vi "MCP23S17 Read REG.vi"(8 "error in (no error)":errorcluster, 10 "Addr":T1 items=["Addr-0"=0, "Addr-1"=4, "Addr-2"=2, "Addr-3"=6, "Addr-4"=1, "Addr-5"=5, "Addr-6"=3, "Addr-7"=7], 11 "handle":u32 format="%08x") -> (0 "error out":errorcluster, 1 "REG B":u16, 2 "REG A":u16, 3 "handle out":u32, 5 "buffer out B":string, 7 "buffer out A":string)   [LabVIEW 2018]
uses:
  PROJEKT/NIKO/Labview/Niko V4/FTDI SPI/Ctl/Sub Addr.ctl
  PROJEKT/NIKO/Labview/Niko V6_A/FTDI SPI/libMPSSE-SPI.lvlib
panel:
  in  "Array U8 2":u8[](array[numeric])=[64, 18, 0, 128, 0, 0, 0, 0, 0, 0] format="%x"
  out "string":string
  in  "Array U8":u8[](array[numeric])=[64, 18, 0, 128, 0, 0, 0, 0, 0, 0] format="%x"
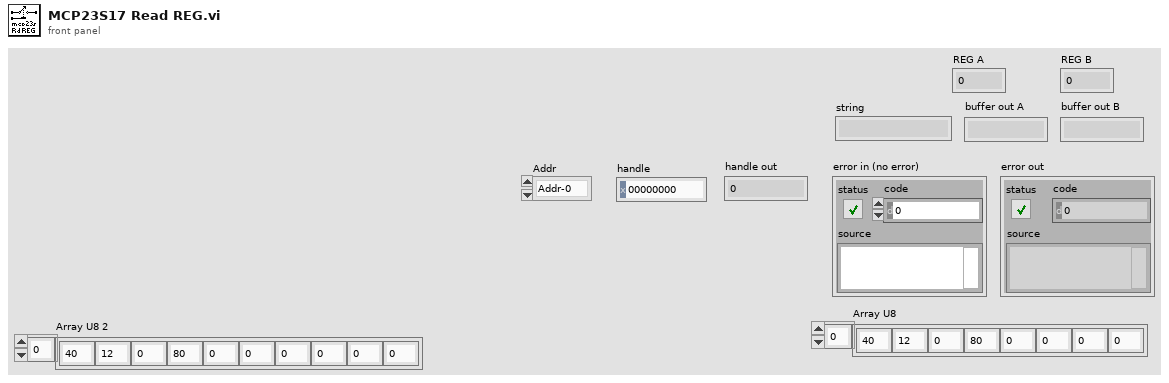
[diagram p1: front panel]
types:
  T1 = typedef "Sub Addr.ctl" = u16
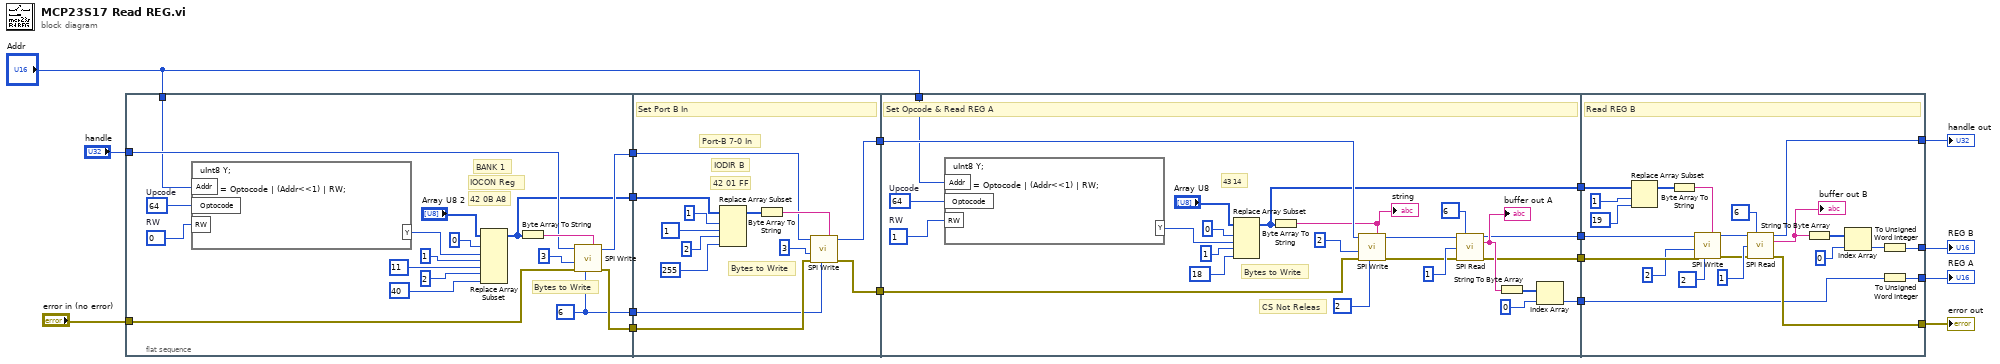
[diagram p0: block diagram]
diagram:
  n1 = flat-sequence {
    tunnel: [w20] -> w7
    tunnel: [w24] -> w6
    tunnel: "handle" -> [w23]
    tunnel: "Addr" -> [w22]
    tunnel: "error in (no error)" -> [w21]
    tunnel: [w19] -> w2
    tunnel: [w18] -> w1
    tunnel: [w41] -> w9
    tunnel: [w40] -> w8
    tunnel: w7 -> [w39]
    tunnel: w6 -> [w38]
    tunnel: w2 -> [w37]
    tunnel: w1 -> [w36]
    tunnel: [w53] -> w16
    tunnel: [w52] -> w15
    tunnel: [w51] -> w14
    tunnel: [w50] -> w13
    tunnel: w9 -> [w68]
    tunnel: w8 -> [w65]
    tunnel: "Addr" -> [w49]
    tunnel: [w92] -> w17
    tunnel: [w91] -> w12
    tunnel: w16 -> [w86]
    tunnel: w15 -> [w82]
    tunnel: w14 -> [w80]
    tunnel: w13 -> [w75]
    tunnel: [w74] -> w11
    tunnel: [w73] -> w10
    frame #0 {
      w35 = u8 64  # Upcode
      w34 = u8 0  # RW
      w18 = u8 6
      # "BANK 1"
      # "IOCON Reg"
      # "Bytes to Write"
      # "42 0B A8"
      n2 = formula code="uInt8 Y;\n      \n    Y = Optocode | (Addr<<1) | RW;"("Addr"=w22, "Optocode"=w35, "RW"=w34) -> ("Y"=w26:u8)
      n3 = Replace Array Subset(array="Array U8 2", new element #1=w26, index #1=0 ("index"), new element #2=u8 11, index #2=u8 1 ("new element/subarray"), new element #3=u8 40, index #3=2 ("index")) -> (w19:u8[])
      n4 = Byte Array To String(unsigned byte array=w19) -> (string=w31:string)
      n5 = call "SPI Write.vi"("buffer"=w31, "options"=w18, "error in (no error)"=w21, "Bytes To Send"=u32 3, "handle"=w23) -> ("error out"=w20:errorcluster, "handle out"=w24:u32)  [unwired: 4 in, 1 out]
    }
    frame #1 {
      # "IODIR B"
      # "Port-B 7-0 In"
      # "Bytes to Write"
      # "42 01 FF"
      # "Set Port B In"
      n6 = Replace Array Subset(array=w37, new element #1=u8 1, index #1=1 ("index"), new element #2=u8 255, index #2=2 ("index")) -> (w45:u8[])
      n7 = Byte Array To String(unsigned byte array=w45) -> (string=w44:string)
      n8 = call "SPI Write.vi"("buffer"=w44, "options"=w36, "error in (no error)"=w39, "Bytes To Send"=u32 3, "handle"=w38) -> ("error out"=w40:errorcluster, "handle out"=w41:u32)  [unwired: 4 in, 1 out]
    }
    frame #2 {
      w61 = u8 64  # Upcode
      w62 = u8 1  # RW
      # "CS Not Releas"
      # "Bytes to Write"
      # "43 14"
      # "Set Opcode & Read REG A"
      n9 = formula code="uInt8 Y;\n      \n    Y = Optocode | (Addr<<1) | RW;"("Addr"=w49, "Optocode"=w61, "RW"=w62) -> ("Y"=w71:u8)
      n10 = Replace Array Subset(array="Array U8", new element #1=w71, index #1=0 ("index"), new element #2=u8 18, index #2=u8 1 ("new element/subarray")) -> (w53:u8[])
      n11 = Byte Array To String(unsigned byte array=w53) -> (string=w67:string)
      "string" <- w67
      n12 = call "SPI Write.vi"("buffer"=w67, "options"=u8 2, "error in (no error)"=w65, "Bytes To Send"=u32 2, "handle"=w68) -> ("error out"=w57:errorcluster, "handle out"=w58:u32)  [unwired: 4 in, 1 out]
      n13 = call "SPI Read.vi"("handle"=w58, "options"=u8 6, "sizeToTransfer"=u32 1, "error in (no error)"=w57) -> ("handle out"=w52:u32, "buffer out"=w54:string, "error out"=w51:errorcluster)  [unwired: 7 in, 2 out]
      "buffer out A" <- w54
      n14 = String To Byte Array(string=w54) -> (unsigned byte array=w55:u8[])
      n15 = Index Array(array=w55, index=0) -> (element=w50:u8)
    }
    frame #3 {
      # "Read REG B"
      n16 = Replace Array Subset(array=w86, new element=u8 19, index=u8 1 ("new element/subarray")) -> (w83:u8[])
      n17 = Byte Array To String(unsigned byte array=w83) -> (string=w81:string)
      n18 = call "SPI Write.vi"("buffer"=w81, "options"=u8 2, "error in (no error)"=w80, "Bytes To Send"=u32 2, "handle"=w82) -> ("error out"=w79:errorcluster, "handle out"=w78:u32)  [unwired: 4 in, 1 out]
      n19 = call "SPI Read.vi"("handle"=w78, "options"=u8 6, "sizeToTransfer"=u32 1, "error in (no error)"=w79) -> ("handle out"=w91:u32, "buffer out"=w90:string, "error out"=w92:errorcluster)  [unwired: 7 in, 2 out]
      "buffer out B" <- w90
      n20 = String To Byte Array(string=w90) -> (unsigned byte array=w89:u8[])
      n21 = Index Array(array=w89, index=0) -> (element=w87:u8)
      n22 = To Unsigned Word Integer(number=w87) -> (unsigned 16bit integer=w73:u16)
      n23 = To Unsigned Word Integer(number=w75) -> (unsigned 16bit integer=w74:u16)
    }
  }
  "error out" <- w17
  "handle out" <- w12
  "REG A" <- w11
  "REG B" <- w10
